vi "configureIntegrationTime.vi"(8 "error in (no error)":errorcluster, 11 "ElectrometerController in":refnum<class "ElectrometerController.lvclass">) -> (0 "error out":errorcluster, 2 "IntegrationTime":dbl=0.002, 3 "ElectrometerController out":refnum<class "ElectrometerController.lvclass">)   [LabVIEW 2016, in "ElectrometerController.lvclass"]
uses:
  ElectrometerController.lvclass
  Electrometer/State/ElectrometerState.lvclass
  Electrometer/Electrometer.lvclass
  ElectrometerConfiguration/ElectrometerInternalConfiguration.lvclass
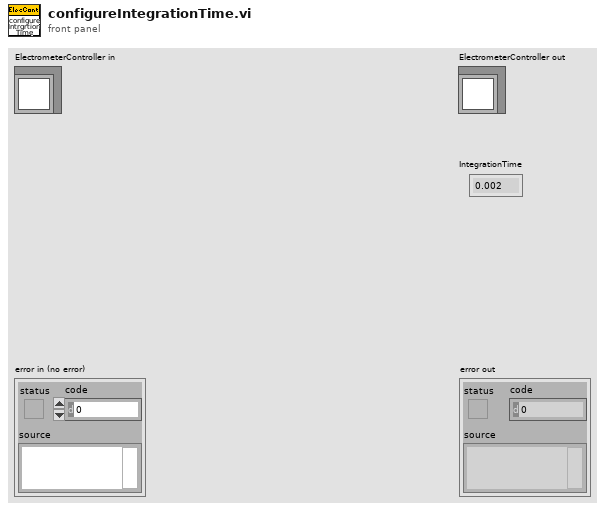
[diagram p1: front panel]
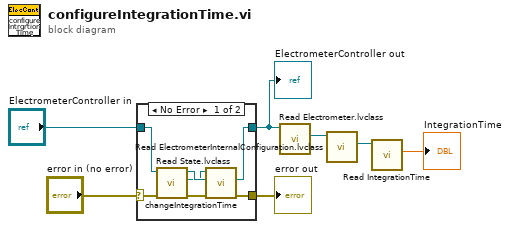
[diagram p0: block diagram]
diagram:
  n1 = case shown="No Error" "error in (no error)" {
    selector: "error in (no error)" -> [w13 w16]
    tunnel: [w11 w16] -> w6
    tunnel: [w12 w15] -> w3
    tunnel: "ElectrometerController in" -> [w14 w15]
    frame No Error {
      n2 = call-dynamic "Read State.lvclass.vi"("error in (no error)"=w13, "ElectrometerController in"=w14) -> ("error out"=w8:errorcluster, "ElectrometerState"=w9:refnum<class "ElectrometerState.lvclass">, "ElectrometerController out"=w10:refnum<class "ElectrometerController.lvclass">)  [unwired: 7 in]
      n3 = call-dynamic "changeIntegrationTime.vi"("error in (no error)"=w8, "ElectrometerController in"=w10, "ElectrometerState in"=w9) -> ("error out"=w11:errorcluster, "ElectrometerController out"=w12:refnum<class "ElectrometerController.lvclass">)  [unwired: 6 in, 1 out]
    }
    frame Error {
    }
  }
  "error out" <- w6
  "ElectrometerController out" <- w3
  n4 = call-dynamic "Read Electrometer.lvclass.vi"("ElectrometerController in"=w3) -> ("Electrometer.lvclass"=w4:refnum<class "Electrometer.lvclass">)  [unwired: 8 in, 2 out]
  n5 = call-dynamic "Read ElectrometerInternalConfiguration.lvclass.vi"("Electrometer in"=w4) -> ("ElectrometerInternalConfiguration.lvclass"=w2:refnum<class "ElectrometerInternalConfiguration.lvclass">)  [unwired: 8 in, 2 out]
  n6 = call-dynamic "Read IntegrationTime.vi"("ElectrometerInternalConfiguration in"=w2) -> ("IntegrationTime"=→"IntegrationTime":dbl)  [unwired: 8 in, 2 out]
